vi "Reset Button.vi"(8 "error in (no error)":errorcluster, 10 "Signaling?":bool, 11 "Button in":refnum<class "Button.lvclass">) -> (0 "error out":errorcluster, 3 "Button out":refnum<class "Button.lvclass">)   [LabVIEW 2020, in "Button.lvlib" / "Button.lvclass"]
uses:
  Button.lvclass
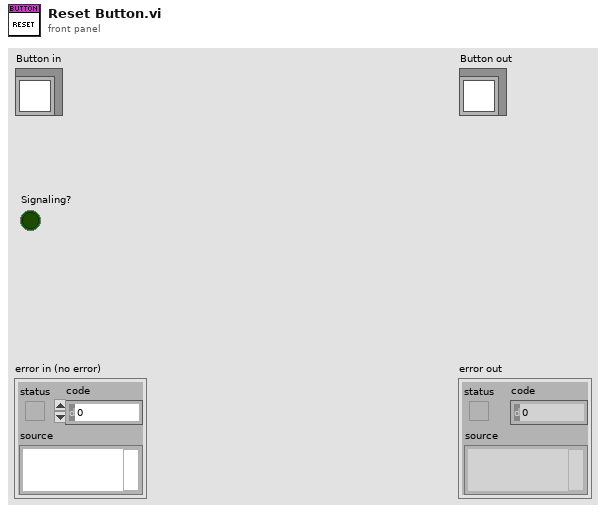
[diagram p1: front panel]
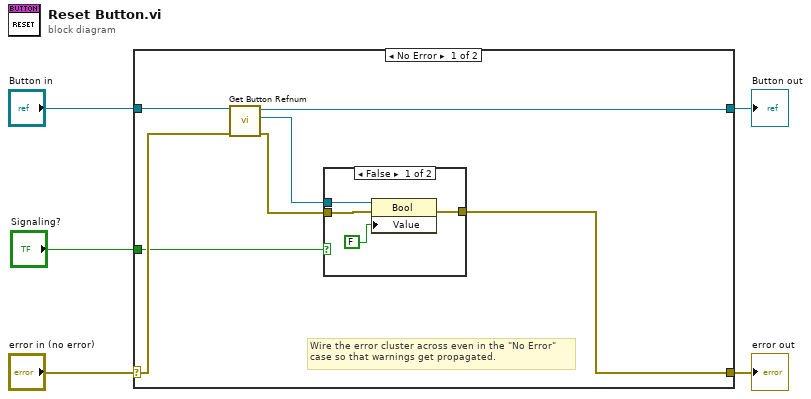
[diagram p0: block diagram]
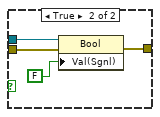
[diagram p2: hidden frame]
diagram:
  n1 = case shown="No Error" "error in (no error)" {
    selector: "error in (no error)" -> [w10 w22]
    tunnel: [w6 w22] -> w4
    tunnel: [w11 w21] -> w2
    tunnel: "Button in" -> [w12 w21]
    tunnel: "Signaling?" -> [w8 _]
    frame No Error {
      # "Wire the error cluster across even in the \"No Error\"\ncase so that warnings get propagated."
      n2 = call "Get Button Refnum.vi"("error in (no error)"=w10, "Button in"=w12) -> ("error out"=w7:errorcluster, "Bool Refnum"=w9:refnum<vi>, "Button out"=w11:refnum<class "Button.lvclass">)  [unwired: 7 in]
      n3 = case shown="False" w8 {
        tunnel: w9 -> [w16 w20]
        tunnel: w7 -> [w15 w19]
        tunnel: [w14 w18] -> w6
        frame False {
          n4 = property class="Bool"(reference=w16, error in=w15, "Value"=FALSE) -> (error out=w14:errorcluster)  [unwired: 1 out]
        }
        frame True {
          n5 = property class="Bool"(reference=w20, error in=w19, "Val(Sgnl)"=FALSE) -> (error out=w18:errorcluster)  [unwired: 1 out]
        }
      }
    }
    frame Error {
    }
  }
  "error out" <- w4
  "Button out" <- w2
